vi "Test Image Write Bad Path.vi"(8 "error in (no error)":errorcluster, 11 "Test Case In":refnum<class "01_Image.lvclass">) -> (0 "error out":errorcluster, 3 "Test Case Out":refnum<class "01_Image.lvclass">)   [LabVIEW 2020, in "test.lvlib" / "01_Image.lvclass"]
uses:
  01_Image.lvclass
  C:/Program Files (x86)/National Instruments/LabVIEW 2026/vi.lib/Astemes/LUnit/Test Case.lvclass
  common/Image Size (Integer).ctl
  <vilib>/Astemes/LUnit/Test Case.lvclass/Test Case.ctl
  image/New Image.vi
  image/New Image (ARGB Preallocated).vi
  image/Copy Array to Image.vi
  image/Copy Array to Image (ARGB).vi
  image/Write Image File (ARGB).vi/9723f547-2605-4a38-b7b5-a8bc0a93fff0.vi
  <vilib>/Astemes/LUnit/Core/LUnit Test Case/Private/Append Fail Result.vi
  <vilib>/Astemes/LUnit/Core/LUnit Test Case/Private/Append Pass Result.vi
  image/New Image (ARGB Preallocated).vi/3321fa97-f432-4e1e-8db9-a0df79aed21b.vi
  image/ARGB Colour to U32 Pixel Value.vi
  <vilib>/Astemes/LUnit/Core/LUnit Test Case/Private/Run In UI.vi
  <vilib>/Utility/error.llb/Clear Errors.vi
  <vilib>/Utility/error.llb/Error Cluster From Error Code.vi
  <vilib>/picture/pixmap.llb/Flatten Pixmap.vi
  common/common.lvlib
  image/image.lvlib
  <vilib>/Astemes/LUnit/Test Case.lvclass
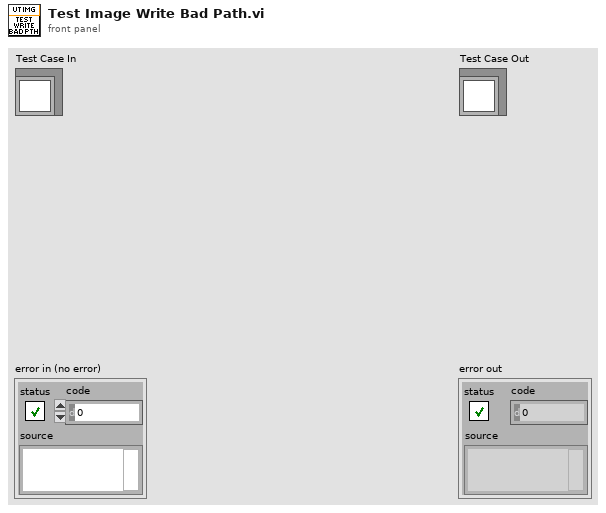
[diagram p1: front panel]
types:
  T1 = typedef "common.lvlib/Image Size (Integer).ctl" = cluster{"Width":u16, "Height":u16}
  T2 = typedef "image.lvlib/ARGB Image.ctl" = refnum<data-value>
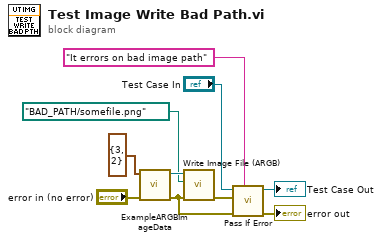
[diagram p0: block diagram]
diagram:
  n1 = call "ExampleARGBImageData.vi"("error in (no error)"="error in (no error)", "Image Size"=T1 {"Width"=3, "Height"=2}) -> ("error out"=w3:errorcluster, "Data Value Reference out"=w5:T2)  [unwired: 6 in, 2 out]
  n2 = call "Write Image File (ARGB).vi"("error in (no error)"=w3, "Filepath in"=path "BAD_PATH/somefile.png", "ARGB Image Source in"=w5) -> ("error out"=w2:errorcluster)  [unwired: 7 in, 1 out]
  n3 = call <vilib>:"Pass If Error.vi"("Description"="It errors on bad image path", "error in (no error)"=w3, "Assert error"=w2, "LUnit Test Case In"="Test Case In") -> ("error out"=→"error out":errorcluster, "LUnit Test Case Out"=→"Test Case Out":refnum<class "01_Image.lvclass">)  [unwired: 6 in]
